vi "Create Parameterized Executive.vi"(4 "File Name":string, 6 "Folder":path, 7 "Attribute Name Blacklist":string[](array[string]), 8 "error in (no error)":errorcluster, 9 "Persistence in":refnum<class "IPersist.lvclass">, 10 "Test Executive":refnum<class "ITest Executive.lvclass">, 11 "Test Executive Ref":refnum<data-value>) -> (0 "error out":errorcluster, 3 "Test Executive Ref out":refnum<data-value>)   [LabVIEW 2019, in "Test Executive.lvlib" / "TestExecutive Ref.lvclass"]
uses:
  <vilib>/gpm_packages/@cs/test-executive/Source/Test Executive/TestExecutive Ref/TestExecutive Ref.lvclass
  <vilib>/gpm_packages/@cs/test-executive/Source/Test Executive/ITestExecutive/ITest Executive.lvclass
  <vilib>/gpm_packages/@cs/persistence/source/IPersist/IPersist.lvclass
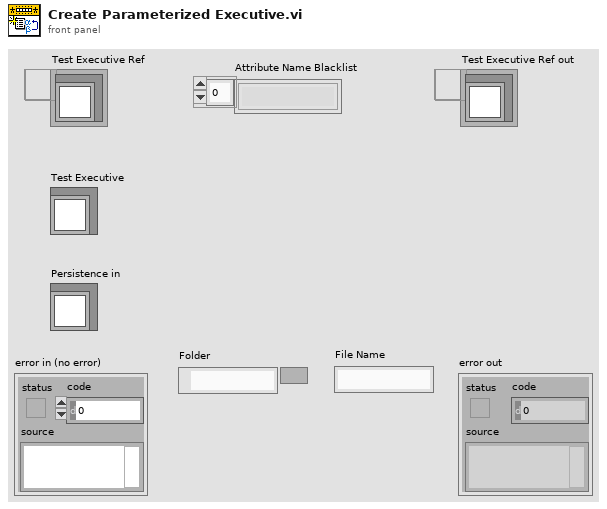
[diagram p1: front panel]
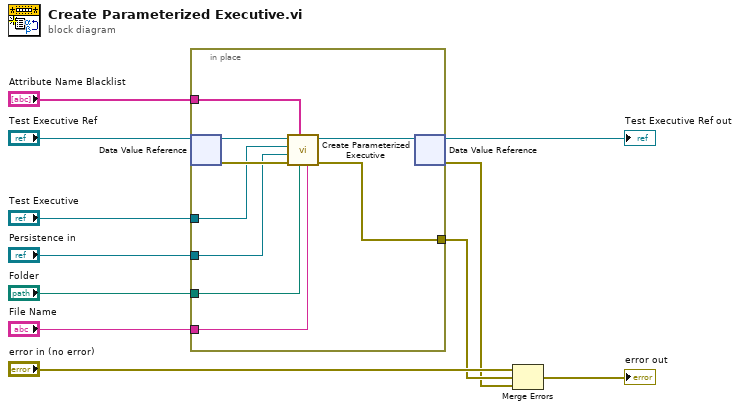
[diagram p0: block diagram]
diagram:
  n1 = in-place {
    in-place-border: [w17] -> w9
    in-place-border: "Test Executive" -> [w16]
    in-place-border: "Persistence in" -> [w15]
    in-place-border: "Folder" -> [w14]
    in-place-border: "File Name" -> [w13]
    in-place-border: "Attribute Name Blacklist" -> [w12]
    n2 = in-place-dvr #1("Test Executive Ref") -> (w20:refnum<class "ITest Executive.lvclass">, w18:errorcluster)
    n3 = call-dynamic "Create Parameterized Executive.vi"("File Name"=w13, "Folder"=w14, "Attribute Name Blacklist"=w12, "error in (no error)"=w18, "Persistence in"=w15, "Test Executive"=w16, "ITest Executive in"=w20) -> ("error out"=w17:errorcluster, "ITest Executive out"=w19:refnum<class "ITest Executive.lvclass">)  [unwired: 3 in]
    n4 = in-place-dvr #1(w19) -> (→"Test Executive Ref out":refnum<data-value>, w8:errorcluster)
  }
  n5 = Merge Errors("error in (no error)", w9, w8) -> (→"error out":errorcluster)
